vi "Create Ball Queue Once.vi"() -> (3 "queue out":refnum<queue>)   [LabVIEW 2019]
uses:
  <vilib>/vision/Image Controls.llb/IMAQ Image.ctl
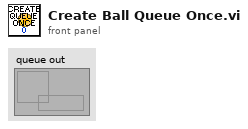
[diagram p1: front panel]
types:
  T1 = typedef "IMAQ Image.ctl" = refnum<image>
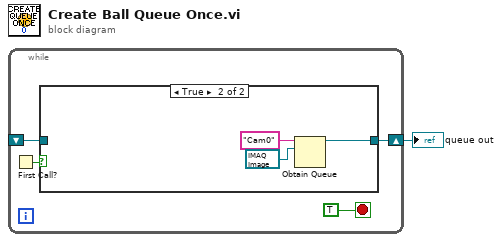
[diagram p0: block diagram]
diagram:
  n1 = while {
    shift-right: [w4] -> w1
    shift-left: _ -> [w3]
    stop <- TRUE stop-if-true
    n2 = First Call?() -> (First Call?: T/F=w5:bool)
    n3 = case shown="True" w5 {
      tunnel: [w6 w7] -> w4
      tunnel: w3 -> [w6 _]
      frame False {
      }
      frame True {
        n4 = Obtain Queue(name (unnamed)="Cam0", element data type=T1 refnum ("Upper Image in")) -> (queue out=w7:refnum<queue>)  [unwired: 3 in, 2 out]
      }
    }
  }
  "queue out" <- w1
